vi "Run 5.vi"(11 "NXT/EV3":T1) -> ()   [LabVIEW 2016]
uses:
  <vilib>/NXT/Subs/LVHSConnector.ctl
  <vilib>/NXT/LegoClasses/BrickReference/BrickReference.lvclass
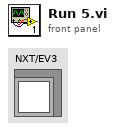
[diagram p1: front panel]
types:
  T1 = typedef "LVHSConnector.ctl" = refnum<class "BrickReference.lvclass">
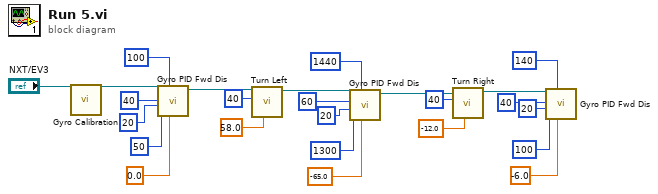
[diagram p0: block diagram]
diagram:
  n1 = call "Gyro Calibration.vi"("NXT/EV3"="NXT/EV3") -> ("NXT/EV3"=w24:T1)  [unwired: 6 in, 2 out]
  n2 = call "Gyro PID Fwd Dis.vi"("Target angle"=sgl 0.0, "Threshold to stop"=100, "Threshold to slow"=50, "Min. speed"=20, "Max. speed"=40, "EV3 in"=w24) -> ("EV3 out"=w18:T1)  [unwired: 5 in]
  n3 = call "Turn Left.vi"("Turning angle"=sgl 58.0, "Motor B (right)"=i8 40, "EV3 in"=w18) -> ("EV3 out"=w10:T1)  [unwired: 8 in]
  n4 = call "Gyro PID Fwd Dis.vi"("Target angle"=sgl -65.0, "Threshold to stop"=1440, "Threshold to slow"=1300, "Min. speed"=20, "Max. speed"=60, "EV3 in"=w10) -> ("EV3 out"=w9:T1)  [unwired: 5 in]
  n5 = call "Turn Right.vi"("Turning angle"=sgl -12.0, "Motor B (right)"=i8 40, "EV3 in"=w9) -> ("EV3 out"=w1:T1)  [unwired: 8 in]
  n6 = call "Gyro PID Fwd Dis.vi"("Target angle"=sgl -6.0, "Threshold to stop"=140, "Threshold to slow"=100, "Min. speed"=20, "Max. speed"=40, "EV3 in"=w1) -> ()  [unwired: 5 in, 1 out]
